vi "System Property Mass Read.vi"(8 "error in (no error)":errorcluster, 11 "System Name":string) -> (0 "error out":errorcluster, 2 "IP Address":string, 3 "Properties Pairs":string[][](array[string]))   [LabVIEW 2016, in "Imager Handler.lvclass"]
uses:
  Imager Handler.lvclass
  <vilib>/nisyscfg/Close (System).vi
  <vilib>/nisyscfg/nisyscfg.lvlib
  <resource>/objmgr/nisysapi.rc
  <resource>/objmgr/motionsysapi.rc
panel:
  out "Benchmark Time (ms)":u32
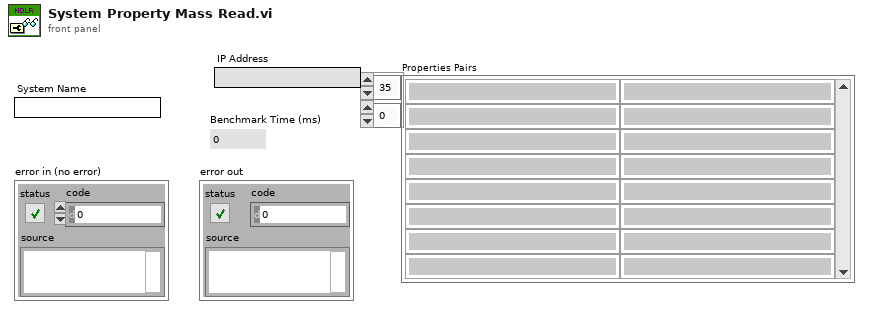
[diagram p1: front panel]
types:
  T1 = typedef "File System.ctl" = i32
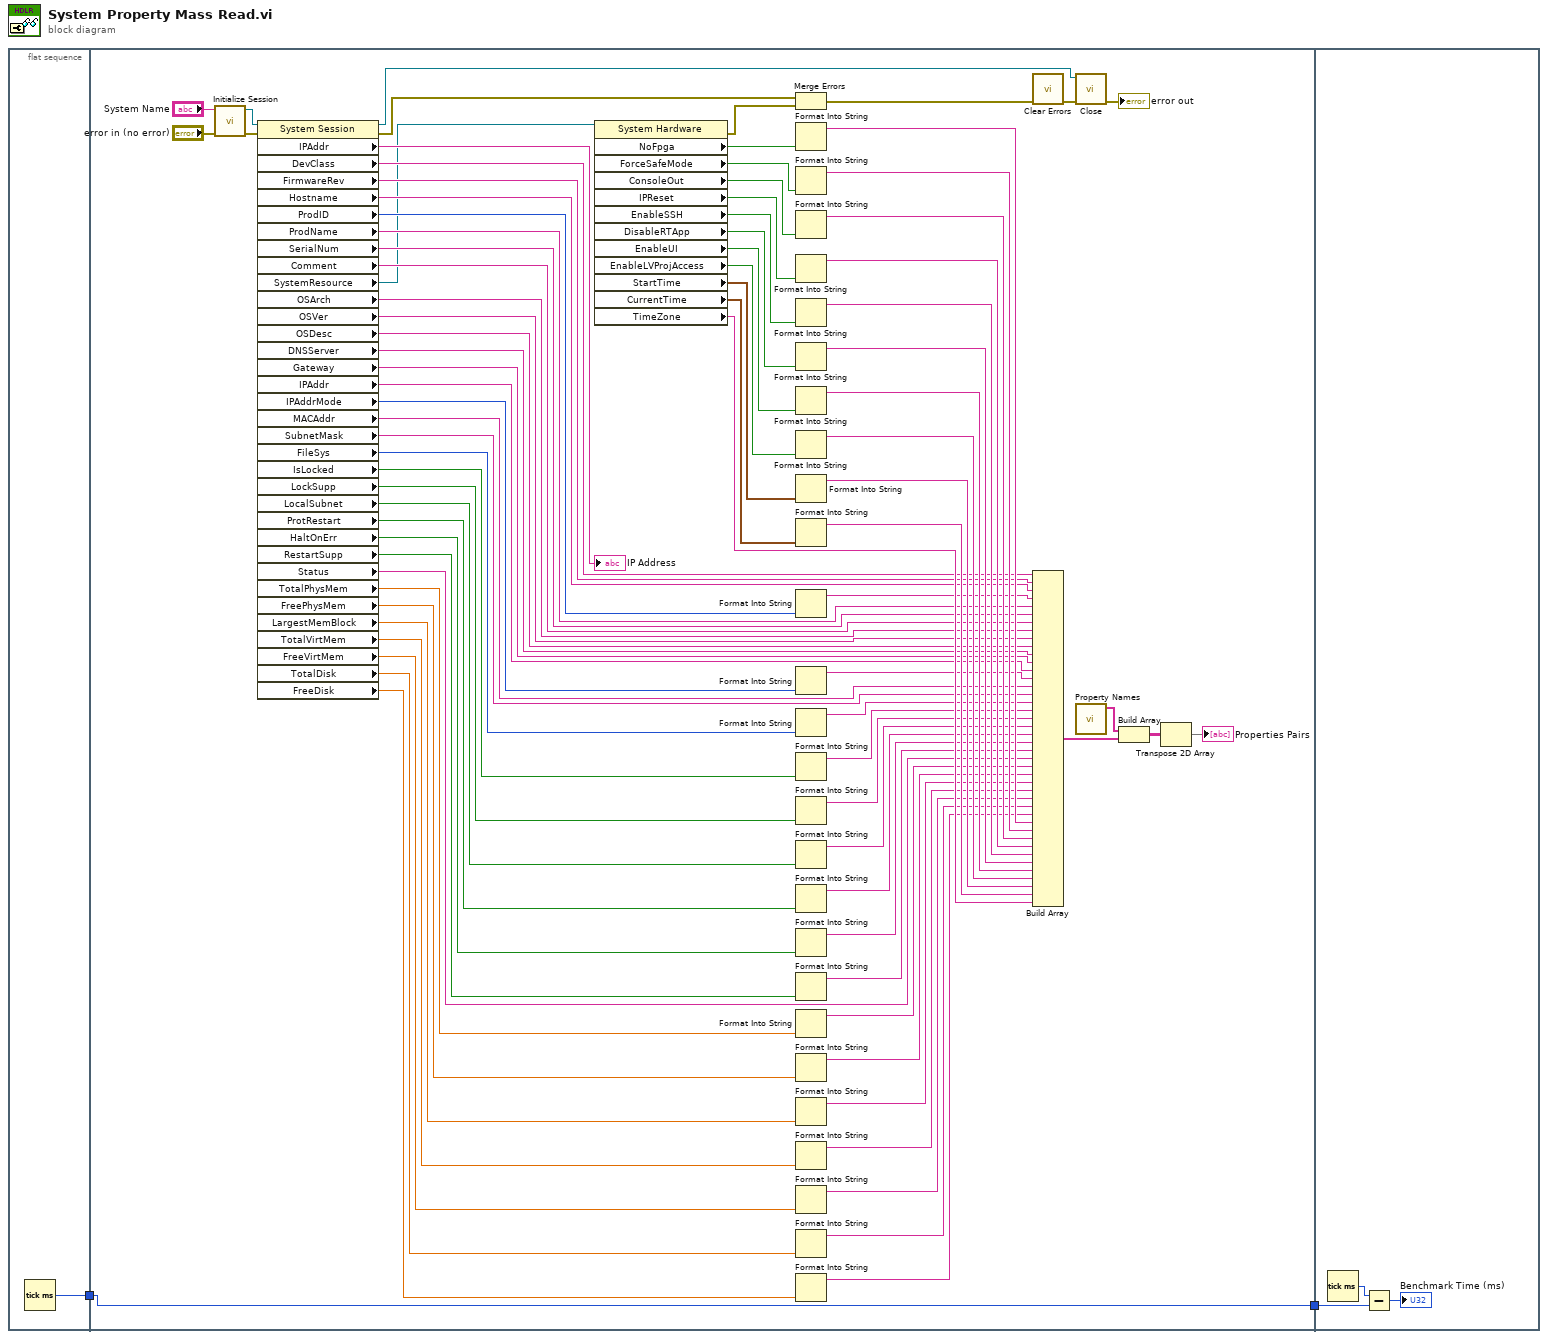
[diagram p0: block diagram]
diagram:
  n1 = flat-sequence {
    tunnel: [w3] -> w1
    tunnel: [w4] -> w2
    tunnel: w1 -> [w4]
    tunnel: w2 -> [w90]
    frame #0 {
      n2 = Tick Count (ms)() -> (millisecond timer value=w3:u32)
    }
    frame #1 {
      n3 = call <vilib>:"Initialize Session.vi"("error in (no error)"="error in (no error)", "Target (localhost)"="System Name") -> ("error out"=w10:errorcluster, "Session out"=w8:refnum<k21>)  [unwired: 8 in]
      n4 = property class="System Session"(reference=w8, error in=w10) -> (reference out=w9:refnum<k21>, error out=w85:errorcluster, "IPAddr"=→"IP Address":string, "DevClass"=w22:string, "FirmwareRev"=w23:string, "Hostname"=w24:string, "ProdID"=w25:i32, "ProdName"=w27:string, "SerialNum"=w28:string, "Comment"=w29:string, "SystemResource"=w11:refnum<k20>, "OSArch"=w30:string, "OSVer"=w31:string, "OSDesc"=w32:string, "DNSServer"=w33:string, "Gateway"=w34:string, "IPAddr"=w35:string, "IPAddrMode"=w36:i32, "MACAddr"=w38:string, "SubnetMask"=w39:string, "FileSys"=w40:T1, "IsLocked"=w42:bool, "LockSupp"=w43:bool, "LocalSubnet"=w44:bool, "ProtRestart"=w45:bool, "HaltOnErr"=w46:bool, "RestartSupp"=w47:bool, "Status"=w54:string, "TotalPhysMem"=w55:dbl, "FreePhysMem"=w56:dbl, "LargestMemBlock"=w57:dbl, "TotalVirtMem"=w58:dbl, "FreeVirtMem"=w59:dbl, "TotalDisk"=w60:dbl, "FreeDisk"=w61:dbl)
      n5 = property class="System Hardware"(reference=w11) -> (error out=w86:errorcluster, "NoFpga"=w14:bool, "ForceSafeMode"=w15:bool, "ConsoleOut"=w16:bool, "IPReset"=w17:bool, "EnableSSH"=w18:bool, "DisableRTApp"=w19:bool, "EnableUI"=w20:bool, "EnableLVProjAccess"=w13:bool, "StartTime"=w12:timestamp, "CurrentTime"=w21:timestamp, "TimeZone"=w79:string)  [unwired: 1 in, 1 out]
      n6 = Merge Errors(w85, w86) -> (w87:errorcluster)
      n7 = Format Into String(w14) -> (resulting string=w69:string)  [unwired: 3 in, 1 out]
      n8 = Format Into String(w15) -> (resulting string=w70:string)  [unwired: 3 in, 1 out]
      n9 = Format Into String(w16) -> (resulting string=w71:string)  [unwired: 3 in, 1 out]
      n10 = Format Into String(w17) -> (resulting string=w72:string)  [unwired: 3 in, 1 out]
      n11 = Format Into String(w18) -> (resulting string=w73:string)  [unwired: 3 in, 1 out]
      n12 = Format Into String(w19) -> (resulting string=w74:string)  [unwired: 3 in, 1 out]
      n13 = Format Into String(w20) -> (resulting string=w75:string)  [unwired: 3 in, 1 out]
      n14 = Format Into String(w13) -> (resulting string=w76:string)  [unwired: 3 in, 1 out]
      n15 = Format Into String(w12) -> (resulting string=w77:string)  [unwired: 3 in, 1 out]
      n16 = Format Into String(w21) -> (resulting string=w78:string)  [unwired: 3 in, 1 out]
      n17 = Format Into String(w25) -> (resulting string=w26:string)  [unwired: 3 in, 1 out]
      n18 = Format Into String(w36) -> (resulting string=w37:string)  [unwired: 3 in, 1 out]
      n19 = Format Into String(w40) -> (resulting string=w41:string)  [unwired: 3 in, 1 out]
      n20 = Format Into String(w42) -> (resulting string=w48:string)  [unwired: 3 in, 1 out]
      n21 = Format Into String(w43) -> (resulting string=w49:string)  [unwired: 3 in, 1 out]
      n22 = Format Into String(w44) -> (resulting string=w50:string)  [unwired: 3 in, 1 out]
      n23 = Format Into String(w45) -> (resulting string=w51:string)  [unwired: 3 in, 1 out]
      n24 = Format Into String(w46) -> (resulting string=w52:string)  [unwired: 3 in, 1 out]
      n25 = Format Into String(w47) -> (resulting string=w53:string)  [unwired: 3 in, 1 out]
      n26 = Format Into String(w55) -> (resulting string=w62:string)  [unwired: 3 in, 1 out]
      n27 = Format Into String(w56) -> (resulting string=w63:string)  [unwired: 3 in, 1 out]
      n28 = Format Into String(w57) -> (resulting string=w64:string)  [unwired: 3 in, 1 out]
      n29 = Format Into String(w58) -> (resulting string=w65:string)  [unwired: 3 in, 1 out]
      n30 = Format Into String(w59) -> (resulting string=w66:string)  [unwired: 3 in, 1 out]
      n31 = Format Into String(w60) -> (resulting string=w67:string)  [unwired: 3 in, 1 out]
      n32 = Format Into String(w61) -> (resulting string=w68:string)  [unwired: 3 in, 1 out]
      n33 = call <vilib>:"Clear Errors.vi"("error in (no error)"=w87) -> ("error out"=w84:errorcluster)  [unwired: 5 in, 1 out]
      n34 = Build Array(w22, w23, w24, w26, w27, w28, w29, w30, w31, w32, w33, w34, w35, w37, w38, w39, w41, w48, w49, w50, w51, w52, w53, w54, w62, w63, w64, w65, w66, w67, w68, w69, w70, w71, w72, w73, w74, w75, w76, w77, w78, w79) -> (w81:string[])
      n35 = call-poly <vilib>:"Close.vi"("error in (no error)"=w84, "Session in"=w9) -> ("error out"=→"error out":errorcluster)  [unwired: 9 in]
      n36 = call "Property Names.vi"() -> ("Property Names"=w80:string[])  [unwired: 11 in]
      n37 = Build Array(w80, w81) -> (w82:string[][])
      n38 = Transpose 2D Array(2D array=w82) -> (transposed array=→"Properties Pairs":string[][])
    }
    frame #2 {
      n39 = Tick Count (ms)() -> (millisecond timer value=w89:u32)
      n40 = Subtract(x=w89, y=w90) -> (x-y=→"Benchmark Time (ms)":u32)
    }
  }
